vi "Configure.vi"(0 "SG Path Power Meter Accessor in":refnum<class "SG Path Accessor.lvclass">, 5 "frequency":dbl=50000000.0, 11 "error in":errorcluster) -> (4 "SG Path Power Meter Accessor out":refnum<class "SG Path Accessor.lvclass">, 15 "error out":errorcluster)   [LabVIEW 2023, in "NI Cal-5501 Power Detector.lvlib" / "SG Path Accessor.lvclass"]
uses:
  SG Path Accessor.lvclass
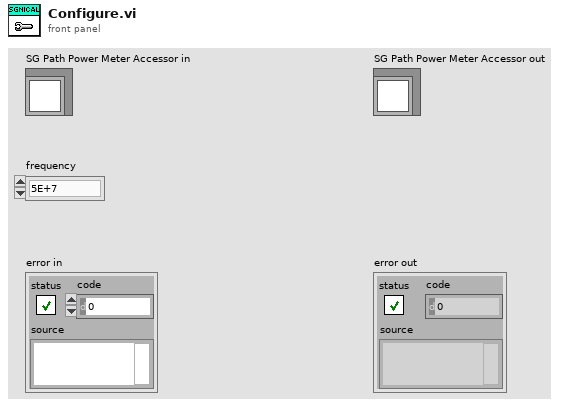
[diagram p1: front panel]
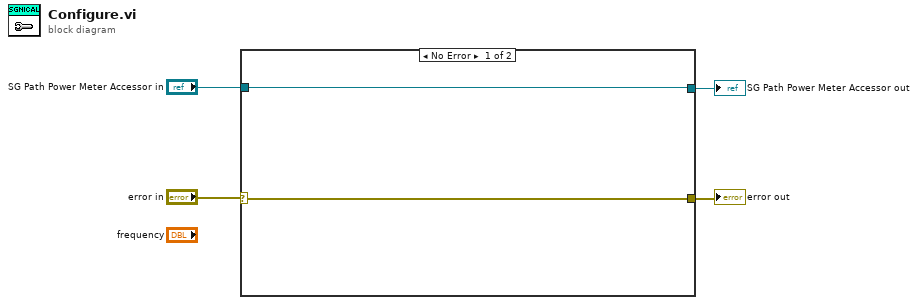
[diagram p0: block diagram]
diagram:
  n1 = case shown="No Error" "error in" {
    selector: "error in" -> [w6 w8]
    tunnel: [w6 w8] -> w3
    tunnel: "SG Path Power Meter Accessor in" -> [w5 w7]
    tunnel: [w5 w7] -> w1
    frame No Error {
    }
    frame Error {
    }
  }
  "error out" <- w3
  "SG Path Power Meter Accessor out" <- w1
